vi "changeRange.vi"(6 "range (V)":dbl, 7 "Device Name":string, 8 "error in (no error)":errorcluster, 9 "Channel (0.1.2.3)":string, 11 "Refnum in":refnum<k21>) -> (0 "error out":errorcluster, 2 "Range":dbl[](array[numeric]), 3 "Refnum out":refnum<k21>)   [LabVIEW 2011]
uses:
  C:/Program Files/National Instruments/LabVIEW 2011/resource/objmgr/daqmx.rc
panel:
  out "Channels":refnum<k21>[](array[refnum])
  out "Range 2":dbl[](array[numeric])
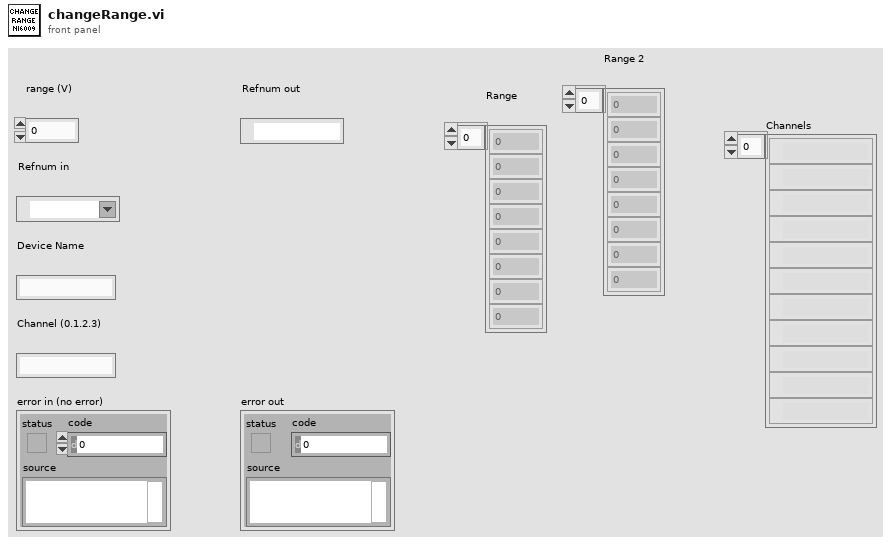
[diagram p1: front panel]
types:
  T1 = typedef "OnOffTypeDef.ctl" = enum16{"off", "on"}
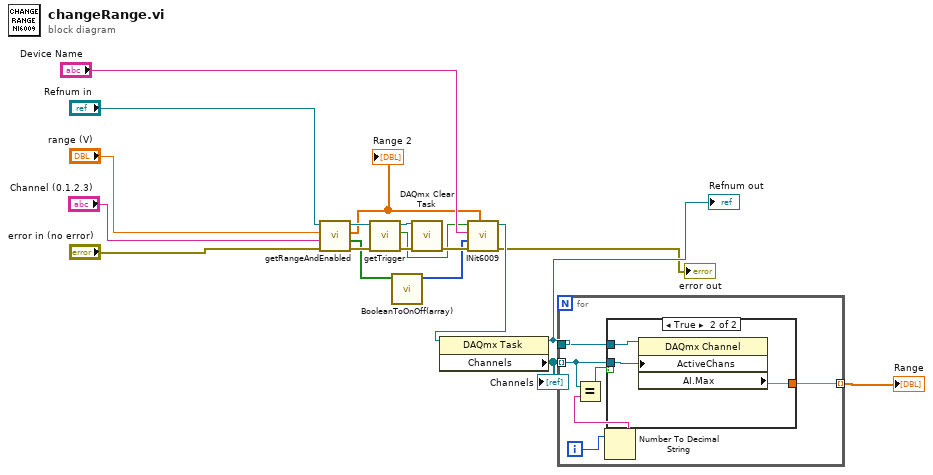
[diagram p0: block diagram]
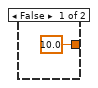
[diagram p2: hidden frame]
diagram:
  n1 = call "getRangeAndEnabled.vi"("error in (no error)"="error in (no error)", "Channel (0.1.2.3)"="Channel (0.1.2.3)", "range (V)"="range (V)", "Refnum in"="Refnum in") -> ("error out"=w10:errorcluster, "Enabled (array)"=w9:bool[], "Range"=w6:dbl[], "Refnum out"=w13:refnum<k21>)  [unwired: 4 in]
  "Range 2" <- w6
  n2 = call "getTrigger.vi"("error in (no error)"=w10, "Refnum in"=w13) -> ("error out"=w11:errorcluster, "triggered"=w7:bool, "Refnum out"=w12:refnum<k21>)  [unwired: 7 in]
  n3 = call "BooleanToOnOff(array).vi"("Enabled (array)"=w9) -> ("Array"=w8:T1[])  [unwired: 10 in]
  n4 = call "DAQmx Clear Task.vi"("task in"=w12, "error in"=w11) -> ("error out"=w14:errorcluster)  [unwired: 13 in]
  n5 = call "INit6009.vi"("Range"=w6, "error in (no error)"=w14, "ChannelEnable"=w8, "DAQmx Device Name"="Device Name", "Trigger"=w7) -> ("error out"=→"error out":errorcluster, "Refnum out"=w5:refnum<k21>)  [unwired: 4 in, 1 out]
  n6 = property class="DAQmx Task"(reference=w5) -> (reference out=w2:refnum<k21>, "Channels"=w4:refnum<k21>[])  [unwired: 1 in, 1 out]
  "Refnum out" <- w2
  "Channels" <- w4
  n7 = for {
    tunnel: w2 -> [w25]
    tunnel: w4 -> [w22] mode=indexing
    tunnel: [w24] -> w3 mode=indexing
    i -> [w23]
    n8 = Number To Decimal String(number=w23) -> (decimal integer string=w21:string)  [unwired: 1 in]
    n9 = Equal?(x=w22, y=w21) -> (x = y?=w20:bool)
    n10 = case shown="True" w20 {
      tunnel: w25 -> [_ w29]
      tunnel: w22 -> [_ w28]
      tunnel: [10.0 ("AI.Max") w27] -> w24
      frame False {
      }
      frame True {
        n11 = property class="DAQmx Channel"(reference=w29, "ActiveChans"=w28) -> ("AI.Max"=w27:dbl)  [unwired: 1 in, 2 out]
      }
    }
  }
  "Range" <- w3
